vi "keccak.host.top.vi"(9 "size":i32, 10 "Bits.in":i32=256, 11 "Data.in":u8[](array[numeric]) format="%.0x") -> (3 "Final.State":u64[](array[numeric]) format="%.0x")   [LabVIEW 2021]
panel:
  out "Numeric 2":u64 format="%.0x"
  out "Debug.State":u64[](array[numeric]) format="%.0x"
  out "Numeric":u64 format="%.0x"
  out "block_size":i32
  out "hash_size":i32
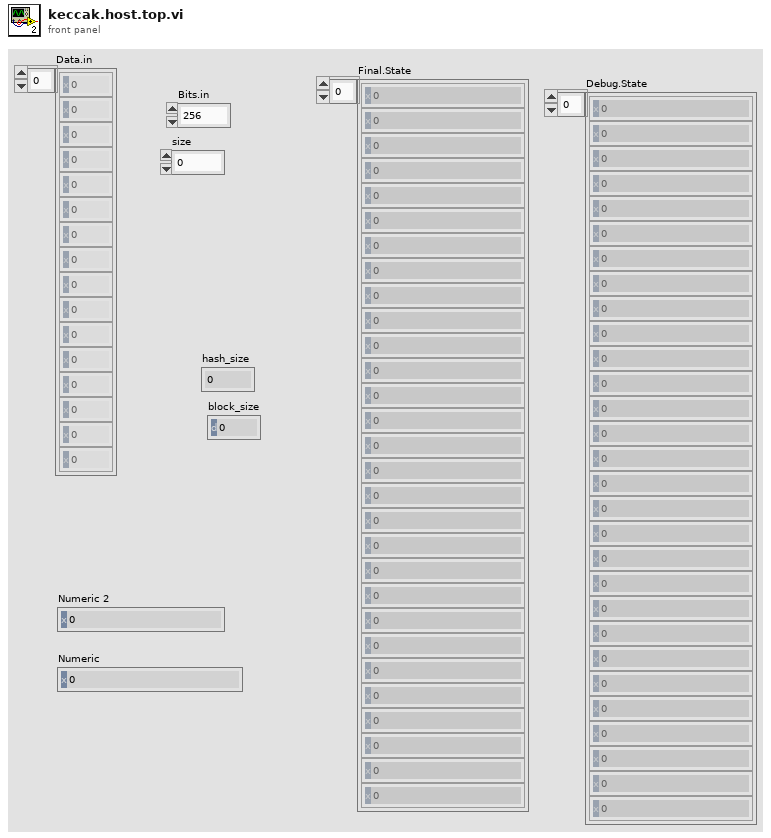
[diagram p1: front panel]
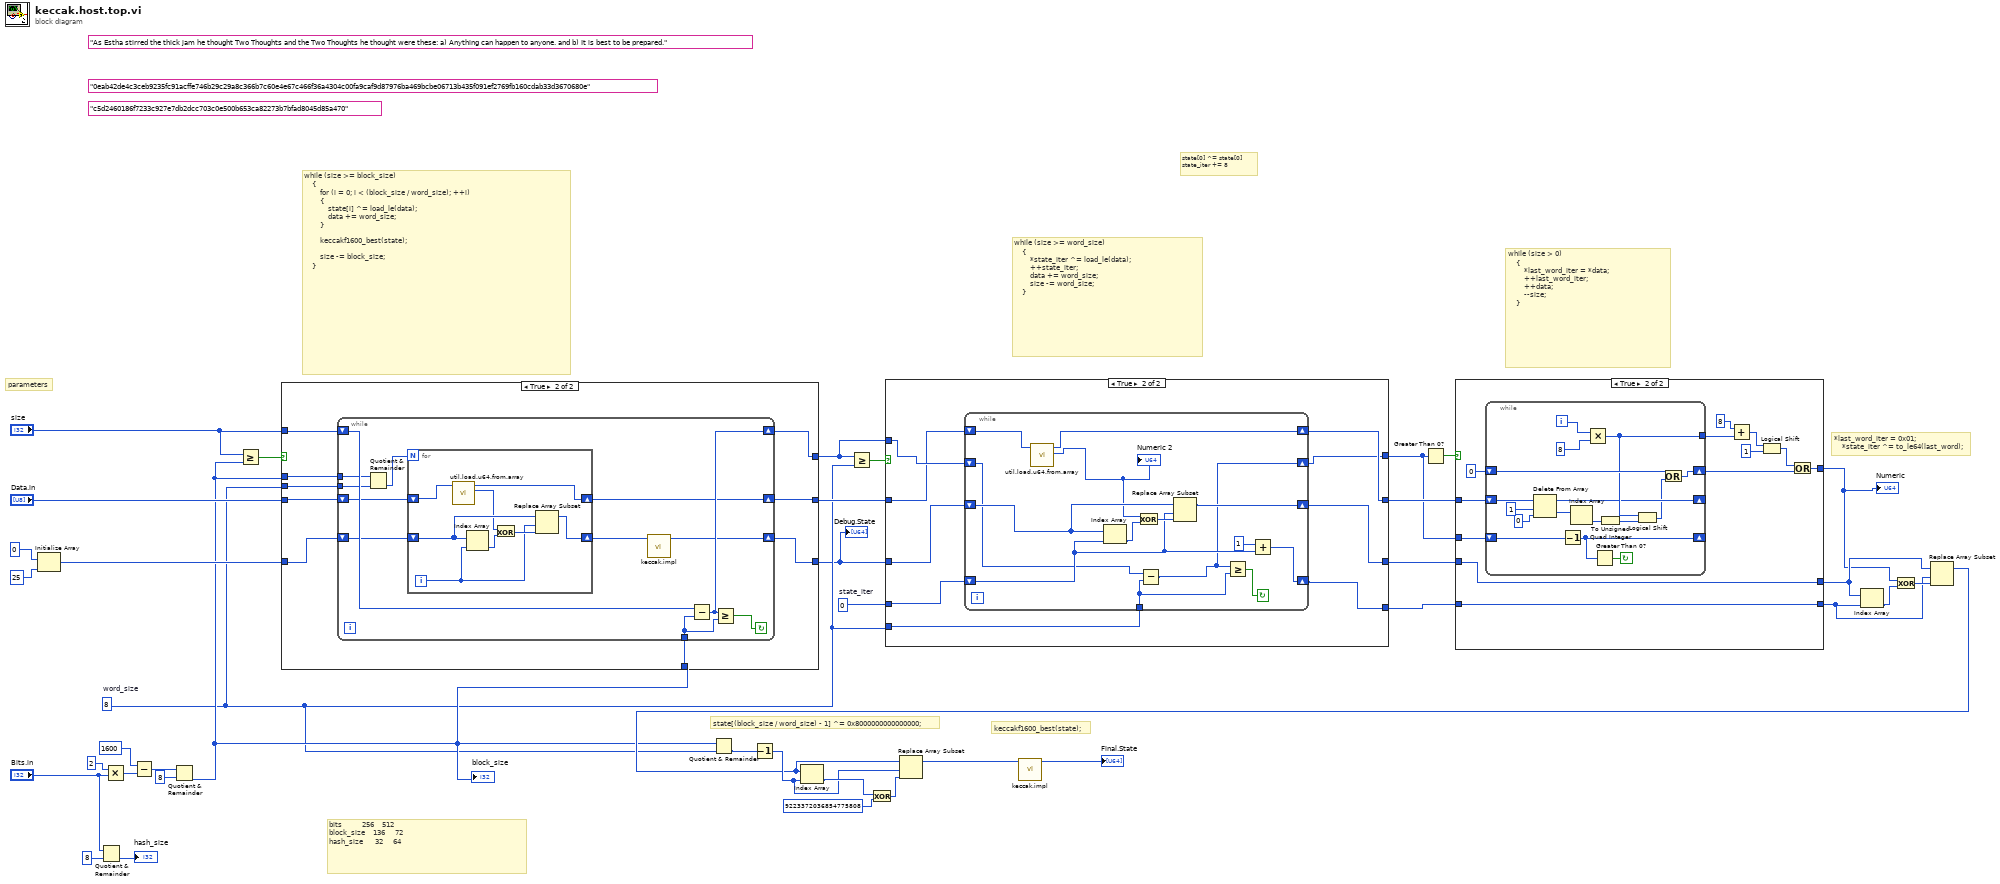
[diagram p0: block diagram]
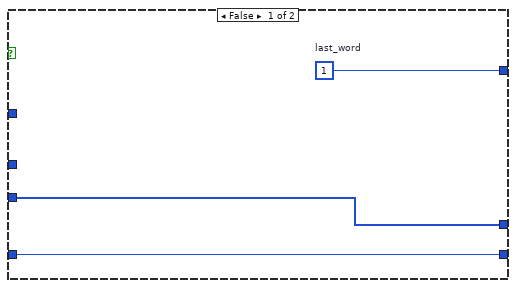
[diagram p4: hidden frame]
diagram:
  w13 = u64 0  # state_iter
  w2 = 8  # word_size
  (unwired) "As Estha stirred the thick jam he thought Two Thoughts and the Two Thoughts he thought were these: a) Anything can happen to anyone. and b) It is best to be prepared."
  (unwired) "0eab42de4c3ceb9235fc91acffe746b29c29a8c366b7c60e4e67c466f36a4304c00fa9caf9d87976ba469bcbe06713b435f091ef2769fb160cdab33d3670680e"
  (unwired) "c5d2460186f7233c927e7db2dcc703c0e500b653ca82273b7bfad8045d85a470"
  # "bits          256    512\nblock_size    136     72\nhash_size      32     64"
  # "state[0] ^= state[0]\nstate_iter += 8"
  # "*last_word_iter = 0x01;\n    *state_iter ^= to_le64(last_word);"
  # "keccakf1600_best(state);"
  # "while (size >= block_size)\n    {\n        for (i = 0; i < (block_size / word_size); ++i)\n        {\n            state[i] ^= load_le(data);\n            data += word_size;\n        }\n\n        keccakf1600_best(state);\n\n        size -= block_size;\n    }"
  # "while (size >= word_size)\n    {\n        *state_iter ^= load_le(data);\n        ++state_iter;\n        data += word_size;\n        size -= word_size;\n    }"
  # "while (size > 0)\n    {\n        *last_word_iter = *data;\n        ++last_word_iter;\n        ++data;\n        --size;\n    }"
  # "state[(block_size / word_size) - 1] ^= 0x8000000000000000;"
  # "parameters"
  n1 = Initialize Array(u64 0, 25 ("dimension size")) -> (w19:u64[])
  n2 = Quotient & Remainder(x="Bits.in", y=8) -> (floor(x/y)=→"hash_size":i32)  [unwired: 1 out]
  n3 = Multiply(x=2, y="Bits.in") -> (x*y=w36:i32)
  n4 = Subtract(x=1600, y=w36) -> (x-y=w34:i32)
  n5 = Quotient & Remainder(x=w34, y=8) -> (floor(x/y)=w3:i32)  [unwired: 1 out]
  "block_size" <- w3
  n6 = Greater Or Equal?(x="size", y=w3) -> (x >= y?=w21:bool)
  n7 = case shown="True" w21 {
    tunnel: [w41 w45] -> w1
    tunnel: w19 -> [w41 w46]
    tunnel: [w42 w49] -> w17
    tunnel: "size" -> [w42 w51]
    tunnel: [w40 w43] -> w7
    tunnel: "Data.in" -> [w40 w44]
    tunnel: w3 -> [_ w50]
    tunnel: w3 -> [_ w48]
    tunnel: w2 -> [_ w47]
    frame False {
    }
    frame True {
      n8 = while {
        tunnel: w50 -> [w61]
        tunnel: w48 -> [w59]
        tunnel: w47 -> [w58]
        shift-right: [w52] -> w45
        shift-left: w46 -> [w56]
        shift-right: [w60] -> w49
        shift-left: w51 -> [w62]
        shift-right: [w54] -> w43
        shift-left: w44 -> [w55]
        stop <- w63 continue-if-true
        n9 = Quotient & Remainder(x=w59, y=w58) -> (floor(x/y)=w57:i32)  [unwired: 1 out]
        n10 = for {
          N: w57 -> [_]
          shift-right: [w71] -> w53
          shift-left: w56 -> [w70]
          shift-right: [w67] -> w54
          shift-left: w55 -> [w68]
          i -> [w64]
          n11 = call "util.load.u64.from.array.vi"("Data.in"=w68) -> ("Numeric"=w66:u64, "Data.out"=w67:u8[])  [unwired: 9 in]
          n12 = Index Array(array=w70, index=w64) -> (element=w69:u64)
          n13 = Exclusive Or(1:w69, 2:w66) -> (0:w65:u64)
          n14 = Replace Array Subset(array=w70, new element=w65, index=w64) -> (w71:u64[])
        }
        n15 = call "keccak.impl.vi"("Array in"=w53) -> ("Array out"=w52:u64[])  [unwired: 10 in]
        n16 = Subtract(x=w62, y=w61) -> (x-y=w60:i32)
        n17 = Greater Or Equal?(x=w60, y=w61) -> (x >= y?=w63:bool)
      }
    }
  }
  "Debug.State" <- w1
  n18 = Quotient & Remainder(x=w3, y=w2) -> (floor(x/y)=w29:i32)  [unwired: 1 out]
  n19 = Decrement(x=w29) -> (x-1=w24:i32)
  n20 = Greater Or Equal?(x=w17, y=w2) -> (x >= y?=w20:bool)
  n21 = case shown="True" w20 {
    tunnel: [w75 w82] -> w6
    tunnel: w1 -> [w75 w83]
    tunnel: [w74 w76] -> w8
    tunnel: w17 -> [w74 w84]
    tunnel: [w73 w78] -> w16
    tunnel: w7 -> [w73 w79]
    tunnel: [w72 w77] -> w14
    tunnel: w13 -> [w72 w81]
    tunnel: w2 -> [_ w80]
    frame False {
    }
    frame True {
      n22 = while {
        shift-right: [w95] -> w82
        shift-left: w83 -> [w94]
        shift-right: [w92] -> w77
        shift-left: w81 -> [w93]
        shift-right: [w89] -> w76
        shift-left: w84 -> [w90]
        tunnel: w80 -> [w88]
        shift-right: [w85] -> w78
        shift-left: w79 -> [w87]
        stop <- w98 continue-if-true
        n23 = call "util.load.u64.from.array.vi"("Data.in"=w87) -> ("Numeric"=w86:u64, "Data.out"=w85:u8[])  [unwired: 9 in]
        "Numeric 2" <- w86
        n24 = Index Array(array=w94, index=w93) -> (element=w96:u64)
        n25 = Exclusive Or(1:w96, 2:w86) -> (0:w97:u64)
        n26 = Subtract(x=w90, y=w88) -> (x-y=w89:i32)
        n27 = Replace Array Subset(array=w94, new element=w97, index=w93) -> (w95:u64[])
        n28 = Greater Or Equal?(x=w89, y=w88) -> (x >= y?=w98:bool)
        n29 = Add(x=u64 1, y=w93) -> (x+y=w92:u64)
      }
    }
  }
  n30 = Greater Than 0?(x=w8) -> (x > 0?=w22:bool)
  n31 = case shown="True" w22 {
    tunnel: w6 -> [w101 w103]
    tunnel: [w101 w103] -> w5
    tunnel: w8 -> [_ w113]
    tunnel: w16 -> [_ w112]
    tunnel: w14 -> [w100 w102]
    tunnel: [w99 w104] -> w4
    tunnel: [w100 w102] -> w9
    frame False {
      w99 = u64 1  # last_word
    }
    frame True {
      n32 = while {
        shift-right: [w127] -> _
        shift-left: w113 -> [w129]
        shift-right: [w121] -> w107
        shift-left: u64 0 -> [w122]
        tunnel: [w118] -> w106
        shift-right: [w117] -> _
        shift-left: w112 -> [w120]
        i -> [w123]
        stop <- w128 continue-if-true
        n33 = Delete From Array(array=w120, length=1, index=0) -> (deleted portion=w125:u8[], array with subset deleted=w117:u8[])
        n34 = Decrement(x=w129) -> (x-1=w127:i32)
        n35 = Index Array(array=w125) -> (element=w115:u8)  [unwired: 1 in]
        n36 = Multiply(x=w123, y=8) -> (x*y=w118:i32)
        n37 = Greater Than 0?(x=w127) -> (x > 0?=w128:bool)
        n38 = To Unsigned Quad Integer(1:w115) -> (0:w114:u64)
        n39 = Logical Shift(y=w118, x=w114) -> (x << y=w116:u64)
        n40 = Or(x=w122, y=w116) -> (x .or. y?=w121:u64)
      }
      n41 = Add(x=8 ("y"), y=w106) -> (x+y=w110:i32)
      n42 = Logical Shift(y=w110, x=u64 1) -> (x << y=w108:u64)
      n43 = Or(x=w108, y=w107) -> (x .or. y?=w104:u64)
    }
  }
  "Numeric" <- w4
  n44 = Index Array(array=w5, index=w9) -> (element=w12:u64)
  n45 = Exclusive Or(1:w12, 2:w4) -> (0:w11:u64)
  n46 = Replace Array Subset(array=w5, new element=w11, index=w9) -> (w10:u64[])
  n47 = Index Array(array=w10, index=w24) -> (element=w28:u64)
  n48 = Exclusive Or(1:u64 9223372036854775808, 2:w28) -> (0:w26:u64)
  n49 = Replace Array Subset(array=w10, new element=w26, index=w24) -> (w25:u64[])
  n50 = call "keccak.impl.vi"("Array in"=w25) -> ("Array out"=→"Final.State":u64[])  [unwired: 10 in]
